vi "FullScreen.vi"(8 "error in (no error)":errorcluster, 10 "FullScr":bool, 11 "Window":string) -> (0 "error out":errorcluster)   [LabVIEW 2020, in "WinAPI.lvlib"]
uses:
  C:/Users/dzoni/Documents/NJ/Playground/LV/WinAPI/DLL/WinAPI.dll
  DLL/WinAPI.dll
  WinAPI.lvlib
panel:
  out "RestoreWindow":bool
  out "X 2":i32
  out "Y 2":i32
  out "Y":i32
  out "X":i32
  out "VI Name":string
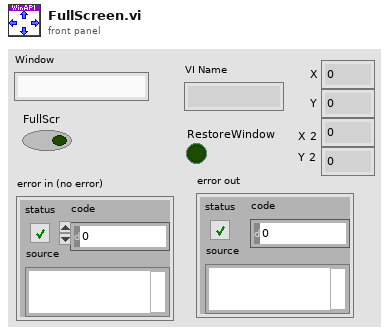
[diagram p1: front panel]
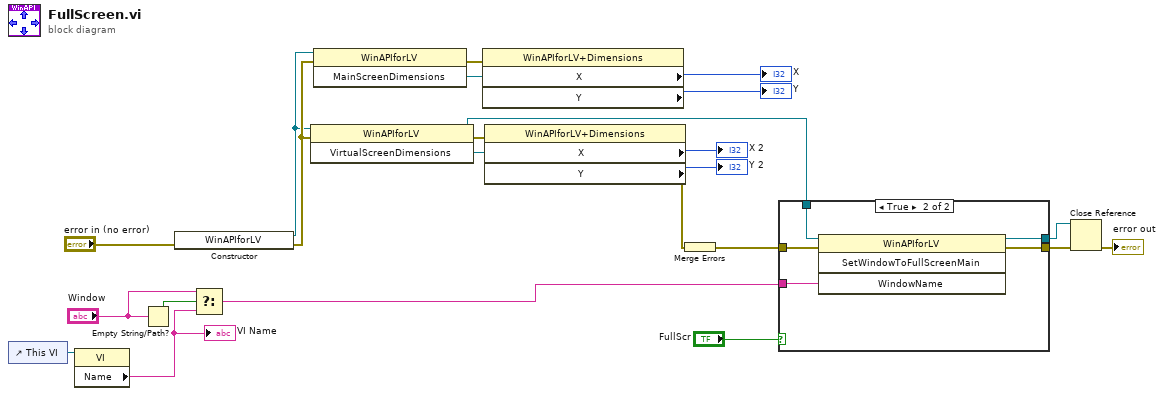
[diagram p0: block diagram]
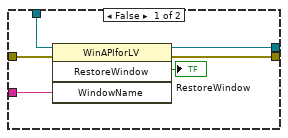
[diagram p2: hidden frame]
diagram:
  n1 = control-ref of="This VI"() -> (w23:refnum<vi>)
  n2 = property class="VI"(reference=w23) -> ("Name"=w2:string)  [unwired: 1 in, 2 out]
  "VI Name" <- w2
  n3 = Empty String/Path?(string/path="Window") -> (empty?=w3:bool)
  n4 = constructor class="WinAPIforLV"(error in="error in (no error)") -> (reference out=w5:refnum<k24>, error out=w6:errorcluster)  [unwired: 2 in, 1 out]
  n5 = Select(t="Window", s=w3, f=w2) -> (s? t:f=w9:string)
  n6 = invoke class="WinAPIforLV" method="VirtualScreenDimensions"(reference=w5, error in=w6) -> (reference out=w7:refnum<k24>, error out=w12:errorcluster, "VirtualScreenDimensions"=w11:refnum<k24>)  [unwired: 1 in]
  n7 = invoke class="WinAPIforLV" method="MainScreenDimensions"(reference=w5, error in=w6) -> (error out=w17:errorcluster, "MainScreenDimensions"=w18:refnum<k24>)  [unwired: 1 in, 1 out]
  n8 = property class="WinAPIforLV+Dimensions"(reference=w18, error in=w17) -> ("X"=→"X":i32, "Y"=→"Y":i32)  [unwired: 2 out]
  n9 = property class="WinAPIforLV+Dimensions"(reference=w11, error in=w12) -> (error out=w8:errorcluster, "X"=→"X 2":i32, "Y"=→"Y 2":i32)  [unwired: 1 out]
  n10 = Merge Errors(w8) -> (w10:errorcluster)
  n11 = case shown="True" "FullScr" {
    tunnel: w9 -> [w28 w34]
    tunnel: w10 -> [w27 w33]
    tunnel: [w25 w31] -> w19
    tunnel: [w26 w32] -> w20
    tunnel: w7 -> [w29 w30]
    frame False {
      n12 = invoke class="WinAPIforLV" method="RestoreWindow"(reference=w29, error in=w27, "WindowName"=w28) -> (reference out=w26:refnum<k24>, error out=w25:errorcluster, "RestoreWindow"=→"RestoreWindow":bool)  [unwired: 1 in, 1 out]
    }
    frame True {
      n13 = invoke class="WinAPIforLV" method="SetWindowToFullScreenMain"(reference=w30, error in=w33, "WindowName"=w34) -> (reference out=w32:refnum<k24>, error out=w31:errorcluster)  [unwired: 1 in, 2 out]
    }
  }
  n14 = Close Reference(reference=w20, error in (no error)=w19) -> (error out=→"error out":errorcluster)
